vi "Camera Data.vi"() -> (0 "Camera Data":T1={"Configuration"={"Settings"={"Pixel clock"=20, "Frame rate"=30.0, "Exposure time"=33.21525, "Master Gain"=0, "Red Gain"=0, "Green Gain"=0, "Blue Gain"=0, "Auto Gain"=FALSE, "White-balance"=FALSE, "Color Correction"=FALSE}}, "Refnums"={"Pixel Clock"=refnum, "Frame Rate"=refnum, "Exposure Time"=refnum, "Master Gain"=refnum, "Red Gain"=refnum, "Green Gain"=refnum, "Blue Gain"=refnum, "Auto Gain"=refnum, "Auto White-balance"=refnum, "Color Correction"=refnum, "Image"=refnum, "Video Button"=refnum, "Instrument Status"=refnum}, "Initialization"={"Connect"=FALSE, "Update Refnums"=FALSE, "Acquiring?"=FALSE}} {"Configuration"."Settings"."Blue Gain" min=0 max=100 scale=0.0..100.0; "Configuration"."Settings"."Green Gain" min=0 max=100 scale=0.0..100.0; "Configuration"."Settings"."Red Gain" min=0 max=100 scale=0.0..100.0; "Configuration"."Settings"."Master Gain" min=0 max=100 scale=0.0..100.0; "Configuration"."Settings"."Exposure time" min=0.101625 max=159.246375 step=0.101625 scale=0.101625..159.246375 scale format="%#.3g"; "Configuration"."Settings"."Frame rate" min=2.7455631699174137 max=6.2675785993528725 step=0.000101625 scale=2.7455631699174137..6.2675785993528725 scale format="%^#_3g"; "Configuration"."Settings"."Pixel clock" min=5 max=43 scale=5.0..43.0})   [LabVIEW 2014]
uses:
  Camera Data.ctl
  Camera Config.ctl
  Camera Settings.ctl
  Camera Refnums.ctl
  support/Instrument Status.ctl
  Camera Initialization.ctl
panel:
  # "LICENSED MATERIALS – PROPERTY OF IBM\nCopyright IBM Corp. 2016,\nALL RIGHTS RESERVED"
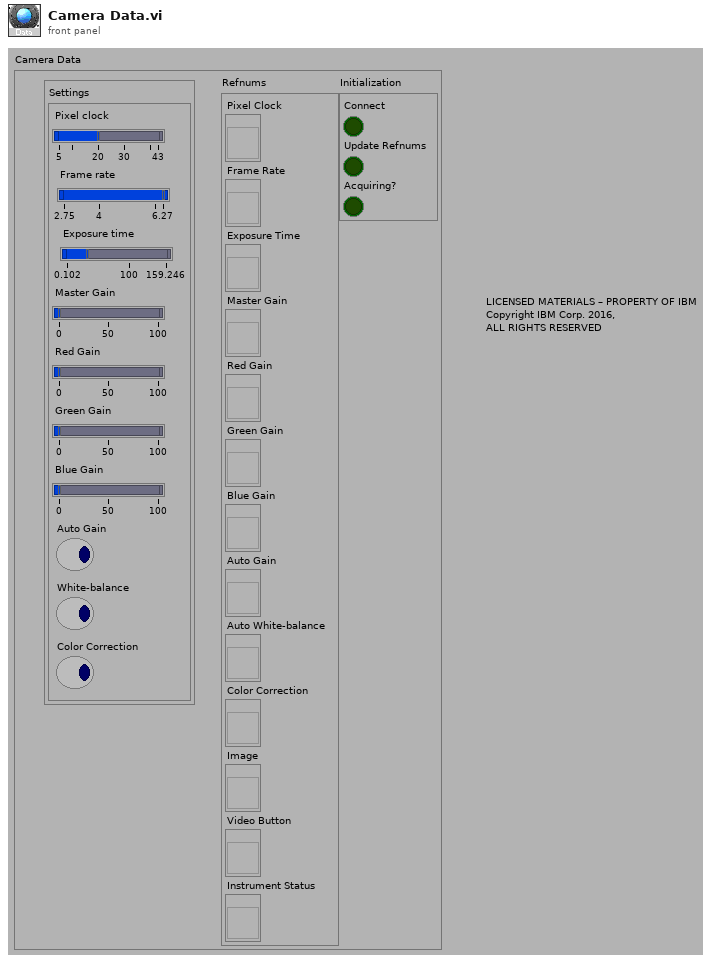
[diagram p1: front panel]
types:
  T1 = typedef "Camera Data.ctl" = cluster{"Configuration":T2, "Refnums":T4, "Initialization":T5}
  T2 = typedef "Camera Config.ctl" = cluster{"Settings":T3}
  T3 = typedef "Camera Settings.ctl" = cluster{"Pixel clock":i32, "Frame rate":dbl, "Exposure time":dbl, "Master Gain":i32, "Red Gain":i32, "Green Gain":i32, "Blue Gain":i32, "Auto Gain":bool, "White-balance":bool, "Color Correction":bool}
  T4 = typedef "Camera Refnums.ctl" = cluster{"Pixel Clock":refnum<vi>, "Frame Rate":refnum<vi>, "Exposure Time":refnum<vi>, "Master Gain":refnum<vi>, "Red Gain":refnum<vi>, "Green Gain":refnum<vi>, "Blue Gain":refnum<vi>, "Auto Gain":refnum<vi>, "Auto White-balance":refnum<vi>, "Color Correction":refnum<vi>, "Image":refnum<vi>, "Video Button":refnum<vi>, "Instrument Status":refnum<vi>}
  T5 = typedef "Camera Initialization.ctl" = cluster{"Connect":bool, "Update Refnums":bool, "Acquiring?":bool}
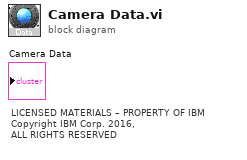
[diagram p0: block diagram]
diagram:
  # "LICENSED MATERIALS – PROPERTY OF IBM\nCopyright IBM Corp. 2016,\nALL RIGHTS RESERVED"
